vi "SetPositioningSpeed.vi"(8 "error in":T1, 11 "speed":i32) -> (0 "error out":T1, 3 "speed out":i32)   [LabVIEW 2016]
doc: "The positioning speed can be defined in both axis 'X' and 'Y' and is provided in nm/s. By passing -2147483648 as input values, the current positioning speed will be read out."
uses:
  Controls/Error_Out.ctl
  Files_ASC500/DLL/ASC500_RemoteControlV27.dll
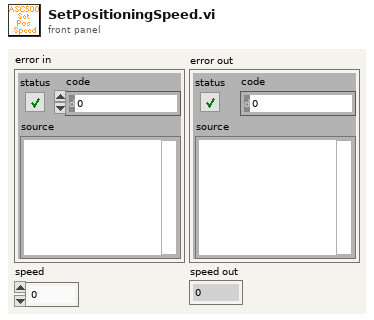
[diagram p1: front panel]
types:
  T1 = typedef "Error_Out.ctl" = errorcluster
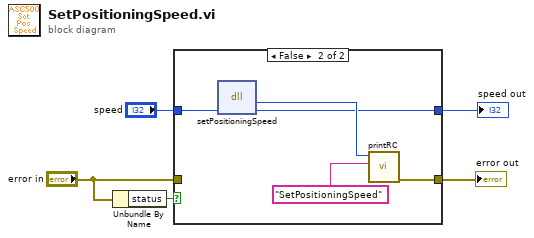
[diagram p0: block diagram]
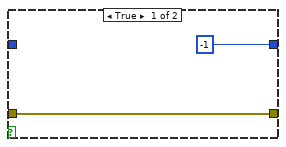
[diagram p2: hidden frame]
diagram:
  n1 = Unbundle By Name("error in") -> ("status"=w4:bool)
  n2 = case shown="False" w4 {
    tunnel: [w7 w12] -> w5
    tunnel: "error in" -> [w7 _]
    tunnel: "speed" -> [_ w9]
    tunnel: [-1 ("Y") w8] -> w1
    frame True {
    }
    frame False {
      n3 = dll-call lib="G:/SCMOperations/Share/ELE/Produkt Information/ASC500/04 Remote Control/02 development versions/2018Nov06/Files_ASC500/DLL/ASC500_RemoteControlV27.dll" fn="setPositioningSpeed"("speed"=w9) -> ("return type"=w11:i32, "speed"=w8:i32)  [unwired: 3 in, 2 out]
      n4 = call "printRC.vi"("additional information"="SetPositioningSpeed", "RC"=w11) -> ("error out"=w12:T1)  [unwired: 9 in]
    }
  }
  "error out" <- w5
  "speed out" <- w1
